vi "sensor_integration_v4.vi"() -> ()   [LabVIEW 2021]
uses:
  controls/sensirion_flow_sensor_data.ctl
panel:
  in  "VISA resource name":refnum<visa-resource-name>
  out "error out":errorcluster
  in  "error in (no error)":errorcluster
  out "VISA resource name out":refnum<visa-resource-name>
  out "retry count":i32
  in  "read byte count (512)":u32=512
  in  "expected num sensors (12)":i32=12
  out "sensor data array":T1[](array[typedef])=[{"flow rate \n(mL/min)"=0.0, "flow val. status"=FALSE, "temp.\n(C)"=0.0, "temp. val status"=FALSE, "air in \nline?"=FALSE, "high \nflow?"=FALSE, "flag. val status"=FALSE}, {"flow rate \n(mL/min)"=0.0, "flow val. status"=FALSE, "temp.\n(C)"=0.0, "temp. val status"=FALSE, "air in \nline?"=FALSE, "high \nflow?"=FALSE, "flag. val status"=FALSE}, {"flow rate \n(mL/min)"=0.0, "flow val. status"=TRUE, "temp.\n(C)"=0.0, "temp. val status"=TRUE, "air in \nline?"=FALSE, "high \nflow?"=FALSE, "flag. val status"=TRUE}, {"flow rate \n(mL/min)"=0.0, "flow val. status"=TRUE, "temp.\n(C)"=0.0, "temp. val status"=TRUE, "air in \nline?"=FALSE, "high \nflow?"=FALSE, "flag. val status"=TRUE}, {"flow rate \n(mL/min)"=0.0, "flow val. status"=TRUE, "temp.\n(C)"=0.0, "temp. val status"=TRUE, "air in \nline?"=FALSE, "high \nflow?"=FALSE, "flag. val status"=TRUE}, {"flow rate \n(mL/min)"=0.0, "flow val. status"=TRUE, "temp.\n(C)"=0.0, "temp. val status"=TRUE, "air in \nline?"=FALSE, "high \nflow?"=FALSE, "flag. val status"=TRUE}, {"flow rate \n(mL/min)"=0.0, "flow val. status"=TRUE, "temp.\n(C)"=0.0, "temp. val status"=TRUE, "air in \nline?"=FALSE, "high \nflow?"=FALSE, "flag. val status"=TRUE}, {"flow rate \n(mL/min)"=0.0, "flow val. status"=TRUE, "temp.\n(C)"=0.0, "temp. val status"=TRUE, "air in \nline?"=FALSE, "high \nflow?"=FALSE, "flag. val status"=TRUE}, {"flow rate \n(mL/min)"=0.0, "flow val. status"=TRUE, "temp.\n(C)"=0.0, "temp. val status"=TRUE, "air in \nline?"=FALSE, "high \nflow?"=FALSE, "flag. val status"=TRUE}, {"flow rate \n(mL/min)"=0.0, "flow val. status"=TRUE, "temp.\n(C)"=0.0, "temp. val status"=TRUE, "air in \nline?"=FALSE, "high \nflow?"=FALSE, "flag. val status"=TRUE}, {"flow rate \n(mL/min)"=0.0, "flow val. status"=TRUE, "temp.\n(C)"=0.0, "temp. val status"=TRUE, "air in \nline?"=FALSE, "high \nflow?"=FALSE, "flag. val status"=TRUE}, {"flow rate \n(mL/min)"=0.0, "flow val. status"=TRUE, "temp.\n(C)"=0.0, "temp. val status"=TRUE, "air in \nline?"=FALSE, "high \nflow?"=FALSE, "flag. val status"=TRUE}] {"temp.\n(C)" scale=20.0..30.0 scale format="%#_3g"; "flow rate \n(mL/min)" scale=0.0..3.0}
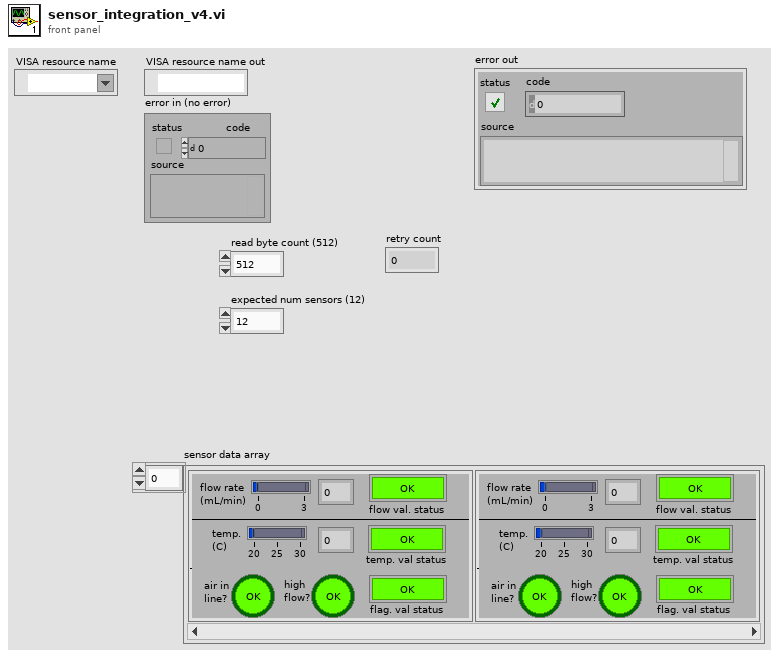
[diagram p1: front panel]
types:
  T1 = typedef "sensirion_flow_sensor_data.ctl" = cluster{"flow rate \n(mL/min)":dbl, "flow val. status":bool, "temp.\n(C)":dbl, "temp. val status":bool, "air in \nline?":bool, "high \nflow?":bool, "flag. val status":bool}
  T2 = typedef "sensirion_flow_sensor_data.ctl" = cluster{"flow rate \n":dbl[unit], "flow val. status":bool, "temperature":dbl[unit], "temp. val status":bool, "air in line?":bool, "high flow?":bool, "flag. val status":bool}
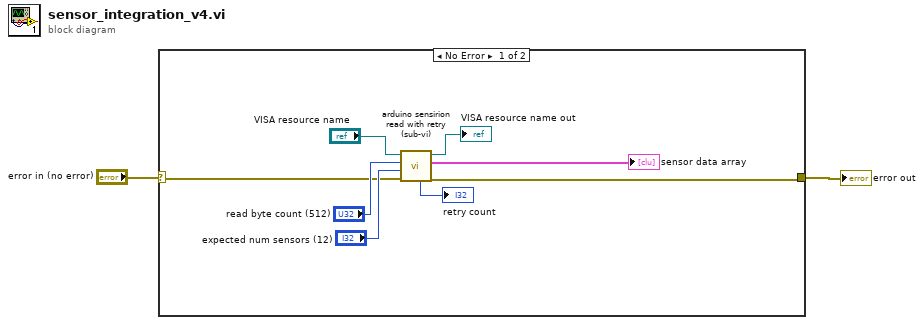
[diagram p0: block diagram]
diagram:
  n1 = case shown="No Error" "error in (no error)" {
    selector: "error in (no error)" -> [w4 w11]
    tunnel: [w5 w11] -> w1
    frame No Error {
      n2 = call "arduino sensirion read with retry (sub-vi).vi"("error in (no error)"=w4, "expected num sensors (12)"="expected num sensors (12)", "read byte count (512)"="read byte count (512)", "VISA resource name"="VISA resource name") -> ("error out"=w5:errorcluster, "sensor data array"=→"sensor data array":T2[], "VISA resource name out"=→"VISA resource name out":refnum<visa-resource-name>, "retry count"=→"retry count":i32)  [unwired: 3 in, 1 out]
    }
    frame Error {
    }
  }
  "error out" <- w1
